vi "Advance past next JSON Value (COPY).vi"(7 "JSON":string, 9 "Offset":i32, 11 "State":T1=enum."Leading Whitespace") -> (1 "index":i32, 2 "Value start":i32, 3 "State":T1=enum."Undefined")   [LabVIEW 2013, in "JSONtext.lvlib"]
uses:
  JSONtext.lvlib
  JSON Value Search.ctl
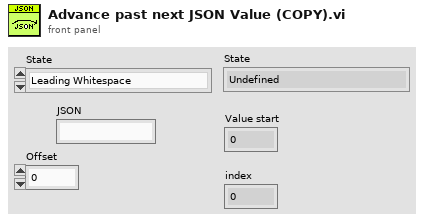
[diagram p1: front panel]
types:
  T1 = typedef "JSONtext.lvlib/JSON Value Search.ctl" = enum16{"Parser Error", "In Object", "In Array", "String", "Number", "Leading Whitespace", "Object end", "Array end", "Value end", "Undefined"}
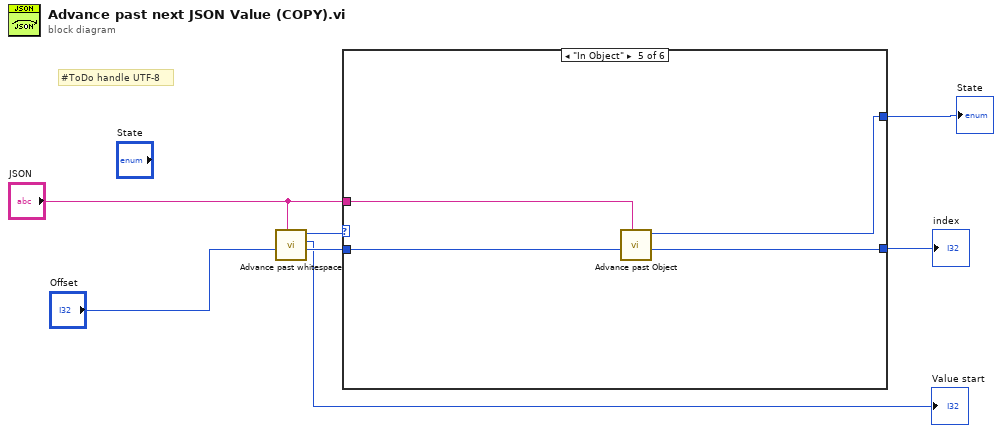
[diagram p0: block diagram]
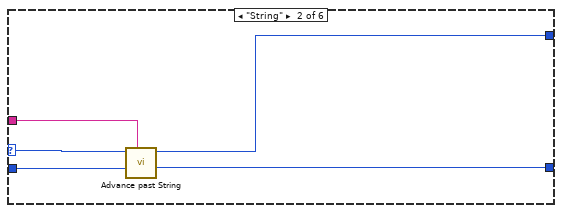
[diagram p3: hidden frame]
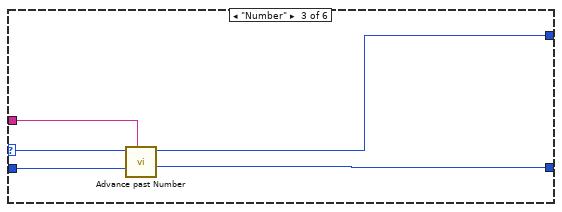
[diagram p4: hidden frame]
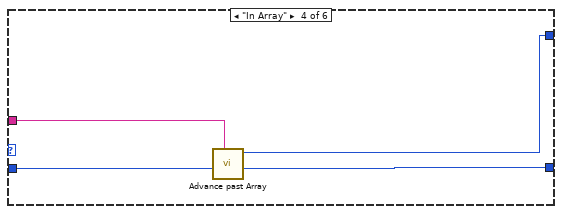
[diagram p5: hidden frame]
diagram:
  # "#ToDo handle UTF-8"
  n1 = call "Advance past whitespace.vi"("JSON"="JSON", "Offset"="Offset") -> ("Offset past match"=w4:i32, "Offset of first non-whitspace"=→"Value start":i32, "State"=w6:T1)  [unwired: 7 in]
  n2 = case shown="\"In Object\"" w6 {
    selector: w6 -> [w8 w13 w18 _ _ w28]
    tunnel: "JSON" -> [_ w14 w19 w20 w24 _]
    tunnel: w4 -> [w9 w12 w17 w21 w27 w29]
    tunnel: [w9 w11 w16 w22 w25 w29] -> w5
    tunnel: [w8 w10 w15 w23 w26 w28] -> w2
    frame "Parser Error", Default {
    }
    frame "String" {
      n3 = call "Advance past String.vi"("JSON"=w14, "Offset"=w12, "State in"=w13) -> ("Offset past match"=w11:i32, "State"=w10:T1)  [unwired: 6 in, 1 out]
    }
    frame "Number" {
      n4 = call "Advance past Number.vi"("JSON"=w19, "Offset (0)"=w17, "Enum in"=w18) -> ("Offset past match"=w16:i32, "Enum out"=w15:T1)  [unwired: 6 in, 1 out]
    }
    frame "In Array" {
      n5 = call "Advance past Array.vi"("JSON"=w20, "Offset"=w21) -> ("Offset past match"=w22:i32, "State"=w23:T1)  [unwired: 7 in, 1 out]
    }
    frame "In Object" {
      n6 = call "Advance past Object.vi"("JSON"=w24, "Offset"=w27) -> ("Offset past Object"=w25:i32, "State"=w26:T1)  [unwired: 8 in]
    }
    frame "Value end" {
      # "null, true, etc."
    }
  }
  "State" <- w2
  "index" <- w5
